vi "UDP Data Link - RTMs - Add Unbound Channels.vi"(8 "error in (no error)":errorcluster, 11 "Node Ptr":u64 format="%.0x") -> (0 "error out":errorcluster)   [LabVIEW 2016, in "UDP-Custom-Device System Explorer.lvlib"]
uses:
  UDP-Custom-Device System Explorer.lvlib
  Types/Channel Data Type.ctl
  <vilib>/NI Veristand/Custom Device API/Custom Device Channel.ctl
  <vilib>/NI Veristand/Custom Device API/Custom Device Channel Type.ctl
  Shared/Constants.vi
  <vilib>/NI Veristand/Custom Device API/Set Item Property (U16).vi
  <vilib>/NI VeriStand/Custom Device API/Custom Device API.lvlib
  Shared/UDP-Custom-Device Shared.lvlib
  <vilib>/NI VeriStand/Custom Device Tools/Custom Device Utility Library/Custom Device Utility Library.lvlib
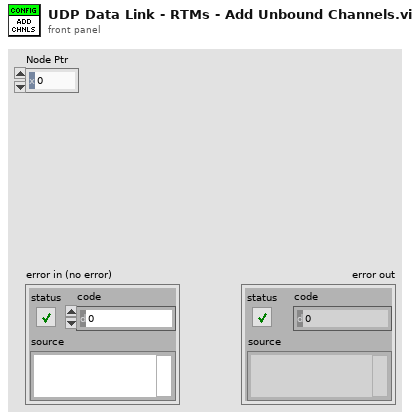
[diagram p1: front panel]
types:
  T1 = typedef "Custom Device API.lvlib/Custom Device Channel.ctl" = cluster{"Type":T2, "Units":string, "Default Value":dbl, "Faultable":bool, "Scalable":bool}
  T2 = typedef "Custom Device API.lvlib/Custom Device Channel Type.ctl" = enum16{"Input", "Output"}
  T3 = typedef "UDP-Custom-Device System Explorer.lvlib/Channel Data Type.ctl" = enum16{"Boolean", "Single"}
  T4 = typedef "Custom Device API.lvlib/Custom Device Item Ref.ctl" = u64
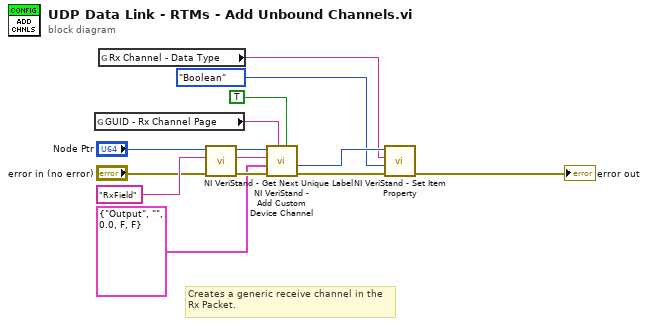
[diagram p0: block diagram]
diagram:
  # "Creates a generic receive channel in the \nRx Packet."
  n1 = global read "Constants.vi" "GUID - Rx Channel Page"() -> (w14:string)
  n2 = global read "Constants.vi" "Rx Channel - Data Type"() -> (w3:string)
  n3 = call <vilib>:"NI VeriStand - Get Next Unique Label.vi"("error in (no error)"="error in (no error)", "Label"="RxField", "Parent Ref in"="Node Ptr") -> ("error out"=w9:errorcluster, "Label out"=w8:string, "Parent Ref dup"=w7:T4)  [unwired: 5 in, 1 out]
  n4 = call <vilib>:"NI VeriStand - Add Custom Device Channel.vi"("Highlight? (F)"=TRUE, "GUID (Default Channel)"=w14, "error in (no error)"=w9, "Channel"=T1 {"Type"=enum."Output", "Units"="", "Default Value"=0.0, "Faultable"=FALSE, "Scalable"=FALSE}, "Channel Name"=w8, "Parent Ref in"=w7) -> ("error out"=w5:errorcluster, "Channel Ref"=w6:T4)  [unwired: 2 in, 2 out]
  n5 = call-poly <vilib>:"NI VeriStand - Set Item Property.vi"("error in (no error)"=w5, "Value"=Channel_Data_Type."Boolean" ("Data Type"), "Property Name"=w3, "Item Ref in"=w6) -> ("error out"=→"error out":errorcluster)  [unwired: 5 in, 2 out]
